vi "ma_In Range with Precision.vi"(8 "precision":i32=6, 9 "low":dbl format="%0.20f", 10 "x":dbl format="%0.20f", 11 "high":dbl format="%0.20f") -> (3 "lo <= x <=  hi?":bool)   [LabVIEW 2020, in "NI_MAPro.lvlib"]
uses:
  NI_MAPro.lvlib
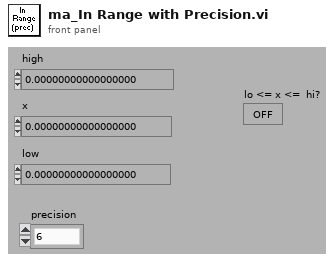
[diagram p1: front panel]
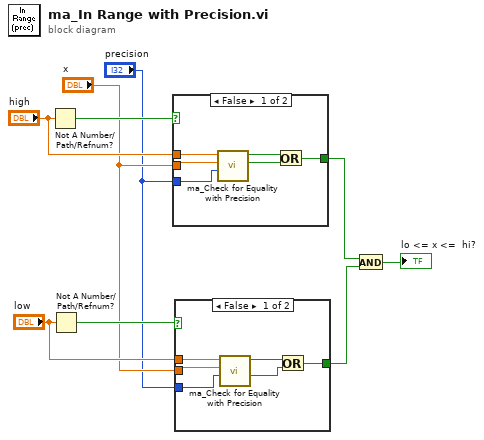
[diagram p0: block diagram]
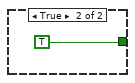
[diagram p2: hidden frame]
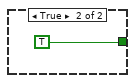
[diagram p3: hidden frame]
diagram:
  n1 = Not A Number/Path/Refnum?(number/path/refnum="high") -> (NaN/Path/Refnum?=w8:bool)
  n2 = Not A Number/Path/Refnum?(number/path/refnum="low") -> (NaN/Path/Refnum?=w5:bool)
  n3 = case shown="False" w8 {
    tunnel: "x" -> [w14 _]
    tunnel: "high" -> [w15 _]
    tunnel: [w11 TRUE] -> w6
    tunnel: "precision" -> [w10 _]
    frame False {
      n4 = call "ma_Check for Equality with Precision.vi"("precision"=w10, "n2"=w14, "n1"=w15) -> ("n1 > n2?"=w12:bool, "equal (within precision)"=w13:bool)  [unwired: 7 out]
      n5 = Or(x=w13, y=w12) -> (x .or. y?=w11:bool)
    }
    frame True {
    }
  }
  n6 = case shown="False" w5 {
    tunnel: "x" -> [w21 _]
    tunnel: "low" -> [w22 _]
    tunnel: [w19 TRUE] -> w2
    tunnel: "precision" -> [w17 _]
    frame False {
      n7 = call "ma_Check for Equality with Precision.vi"("precision"=w17, "n2"=w21, "n1"=w22) -> ("n1 < n2?"=w18:bool, "equal (within precision)"=w20:bool)  [unwired: 7 out]
      n8 = Or(x=w20, y=w18) -> (x .or. y?=w19:bool)
    }
    frame True {
    }
  }
  n9 = And(x=w6, y=w2) -> (x .and. y?=→"lo <= x <=  hi?":bool)
